vi "Gui.vi"() -> ()   [LabVIEW 2013]
uses:
  GlobalStop.vi
  GlobalWrite.vi
  GlobalMFC.vi
  GlobalGraph.vi
  GlobalMFCread.vi
panel:
  in  "TIME_INTERVAL (SECONDS)":dbl=1.0
  out "MFC_OUTPUT":dbl[](array[numeric])
  in  "MFC_INPUT":dbl[](array[numeric])
  out "URAS_OUTPUT_GRAPH":dynamicdata(graph)
  out "EUROTHERM_OUTPUT_GRAPH":dynamicdata(graph)
  in  "?":bool
  in  "EUROTHERM_INPUT":dbl[](array[numeric])
  out "EUROTHERM_OUTPUT":dbl[](array[numeric])
  # "O2"
  # "O2"
  # "CO"
  # "CO"
  # "HE"
  # "HE"
  # "N2"
  # "N2"
  # "CO2"
  # "CO2"
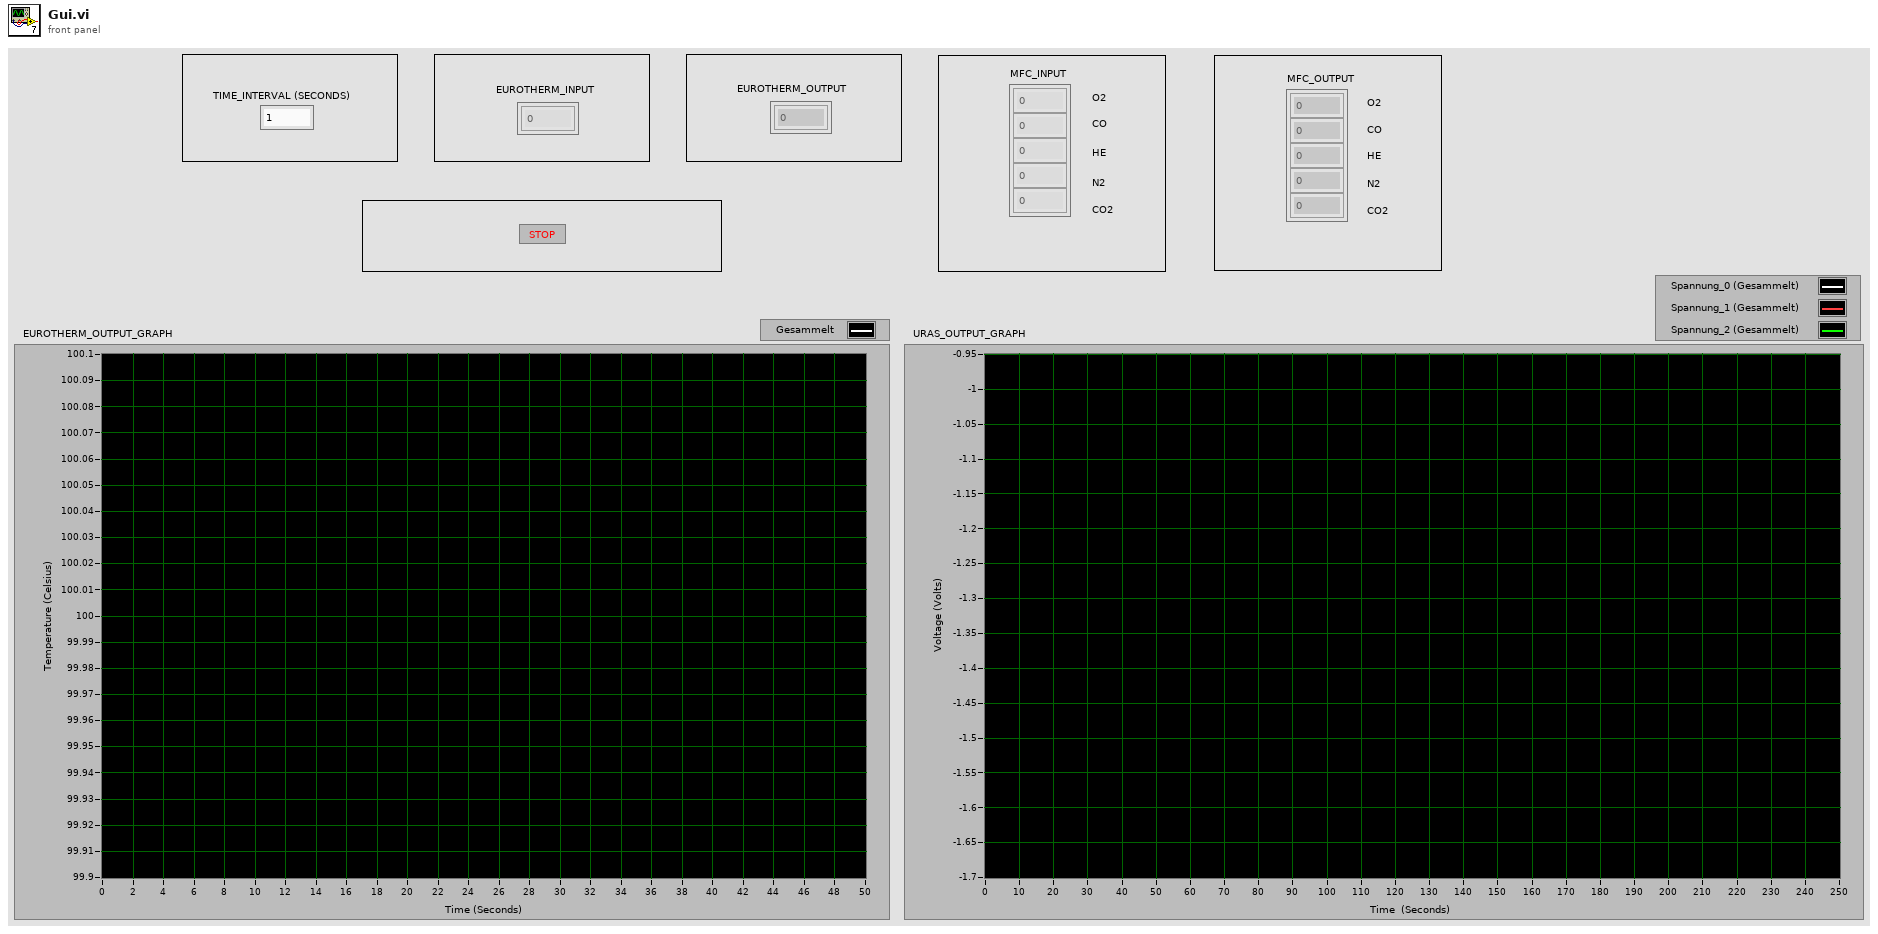
[diagram p1: front panel]
types:
  T1 = enum32{"Invalid", "Standard", "Closed", "Hidden", "Minimized", "Maximized"}
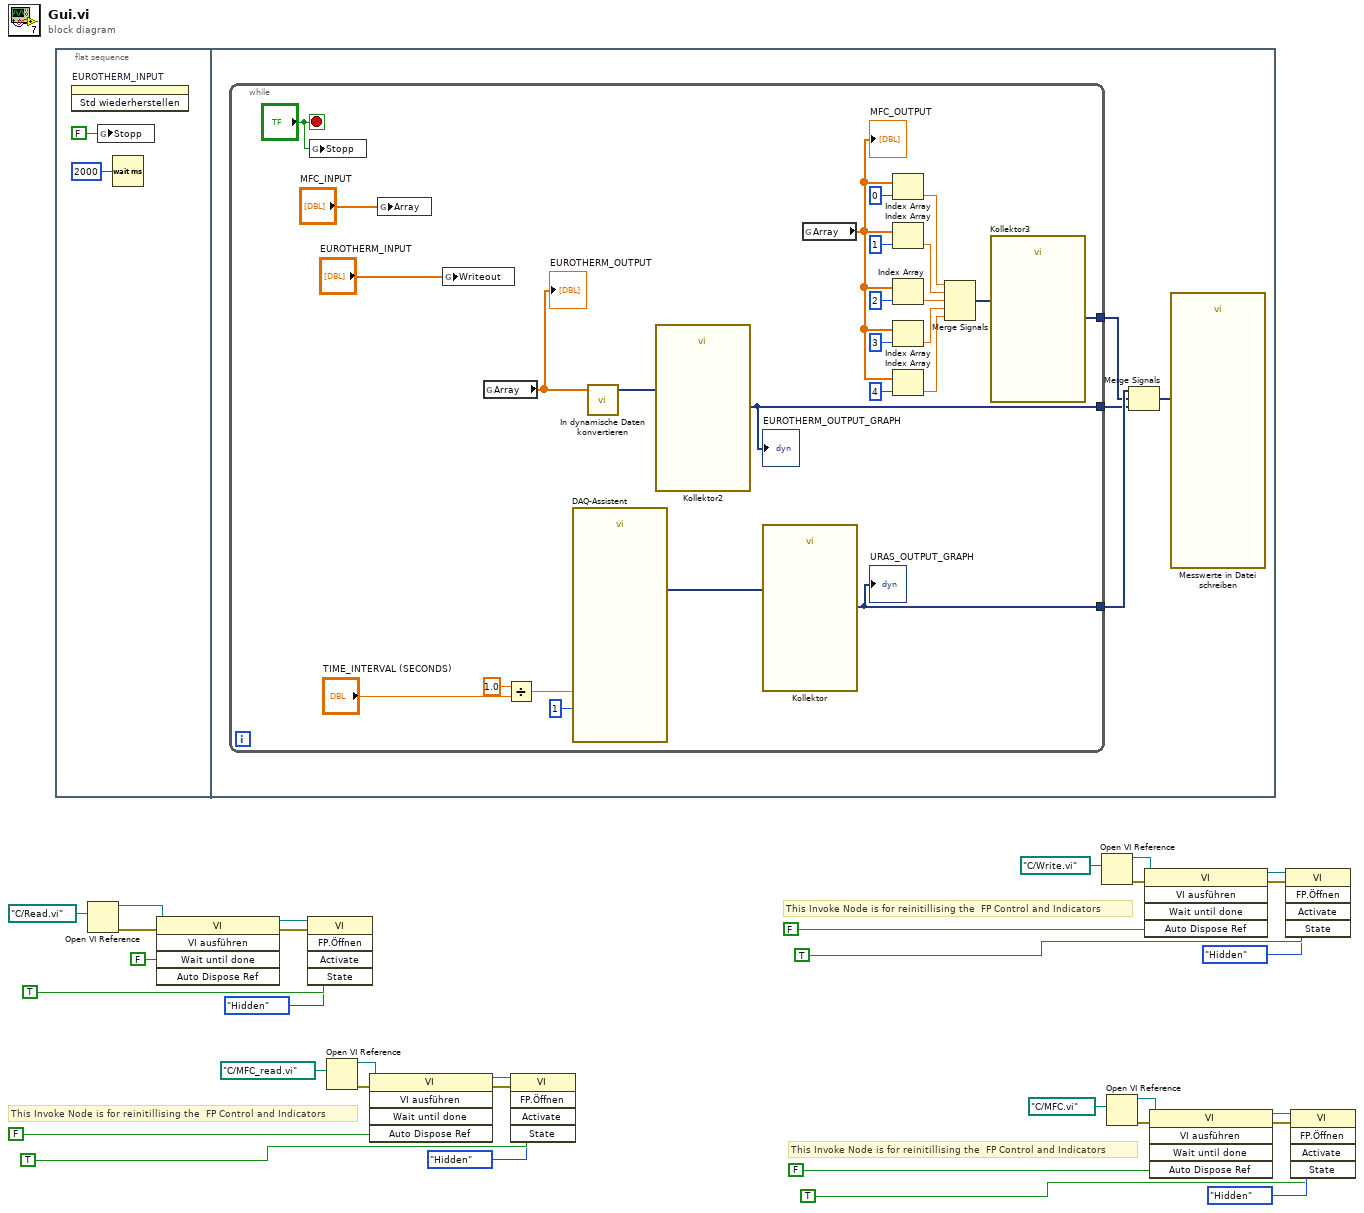
[diagram p0: block diagram]
diagram:
  # "This Invoke Node is for reinitillising the  FP Control and Indicators"
  # "This Invoke Node is for reinitillising the  FP Control and Indicators"
  # "This Invoke Node is for reinitillising the  FP Control and Indicators"
  n1 = flat-sequence {
    frame #0 {
      n2 = invoke on="EUROTHERM_INPUT" class="Arr (strikt)" method="Std wiederherstellen"() -> ()  [unwired: 3 in, 3 out]
      n3 = global write "GlobalStop.vi" "Stopp"(FALSE) -> ()
      n4 = Wait (ms)(milliseconds to wait=u32 2000 ("Zu wartende ms")) -> ()  [unwired: 1 out]
    }
    frame #1 {
      n5 = while {
        tunnel: [w60] -> w37
        tunnel: [w56] -> w35
        tunnel: [w51] -> w36
        stop <- "?" stop-if-true
        n6 = global write "GlobalStop.vi" "Stopp"("?") -> ()
        n7 = global write "GlobalMFC.vi" "Array"("MFC_INPUT") -> ()
        n8 = global write "GlobalWrite.vi" "Writeout"("EUROTHERM_INPUT") -> ()
        n9 = global read "GlobalGraph.vi" "Array"() -> (w50:dbl[])
        "EUROTHERM_OUTPUT" <- w50
        n10 = Divide(x=1.0, y="TIME_INTERVAL (SECONDS)") -> (x/y=w54:dbl)
        n11 = call "DAQ-Assistent"("Rate"=w54, "Sample-Anzahl"=1) -> ("data"=w61:dynamicdata)  [unwired: 14 in, 3 out]
        n12 = call "In dynamische Daten konvertieren"("Array"=w50) -> ("Dynamic Data Type"=w49:dynamicdata)  [unwired: 3 in]
        n13 = call "Kollektor2"("Signals"=w49) -> ("Collected Signals"=w51:dynamicdata)  [unwired: 9 in, 1 out]
        "EUROTHERM_OUTPUT_GRAPH" <- w51
        n14 = call "Kollektor"("Signals"=w61) -> ("Collected Signals"=w60:dynamicdata)  [unwired: 9 in, 1 out]
        "URAS_OUTPUT_GRAPH" <- w60
        n15 = global read "GlobalMFCread.vi" "Array"() -> (w48:dbl[])
        "MFC_OUTPUT" <- w48
        n16 = Index Array(array=w48, index=0 ("Index")) -> (element=w57:dbl)
        n17 = Index Array(array=w48, index=1 ("Index")) -> (element=w42:dbl)
        n18 = Index Array(array=w48, index=2 ("Index")) -> (element=w41:dbl)
        n19 = Index Array(array=w48, index=3 ("Index")) -> (element=w40:dbl)
        n20 = Index Array(array=w48, index=4 ("Index")) -> (element=w39:dbl)
        n21 = Merge Signals(w57, w42, w41, w40, w39) -> (w43:dynamicdata)
        n22 = call "Kollektor3"("Signals"=w43) -> ("Collected Signals"=w56:dynamicdata)  [unwired: 9 in, 1 out]
      }
      n23 = Merge Signals(w37, w35, w36) -> (w38:dynamicdata)
      n24 = call "Messwerte in Datei schreiben"("Signals"=w38) -> ()  [unwired: 16 in, 3 out]
    }
  }
  n25 = Open VI Reference(vi path=path "C:/Read.vi" ("VI-Pfad")) -> (vi reference=w29:refnum<vi>, error out=w28:errorcluster)  [unwired: 5 in]
  n26 = invoke class="VI" method="VI ausführen"(reference=w29, error in=w28, "Wait until done"=FALSE) -> (reference out=w24:refnum<vi>, error out=w23:errorcluster)  [unwired: 2 in, 3 out]
  n27 = invoke class="VI" method="FP.Öffnen"(reference=w24, error in=w23, "Activate"=TRUE ("Aktivieren?"), "State"=T1."Hidden" ("Zustand")) -> ()  [unwired: 1 in, 5 out]
  n28 = Open VI Reference(vi path=path "C:/MFC_read.vi" ("VI-Pfad")) -> (vi reference=w8:refnum<vi>, error out=w7:errorcluster)  [unwired: 5 in]
  n29 = invoke class="VI" method="VI ausführen"(reference=w8, error in=w7, "Wait until done"=FALSE) -> (reference out=w5:refnum<vi>, error out=w4:errorcluster)  [unwired: 2 in, 3 out]
  n30 = invoke class="VI" method="FP.Öffnen"(reference=w5, error in=w4, "Activate"=TRUE ("Aktivieren?"), "State"=T1."Hidden" ("Zustand")) -> ()  [unwired: 1 in, 5 out]
  n31 = Open VI Reference(vi path=path "C:/Write.vi" ("VI-Pfad")) -> (vi reference=w32:refnum<vi>, error out=w31:errorcluster)  [unwired: 5 in]
  n32 = Open VI Reference(vi path=path "C:/MFC.vi" ("VI-Pfad")) -> (vi reference=w10:refnum<vi>, error out=w11:errorcluster)  [unwired: 5 in]
  n33 = invoke class="VI" method="VI ausführen"(reference=w32, error in=w31, "Wait until done"=FALSE) -> (reference out=w20:refnum<vi>, error out=w19:errorcluster)  [unwired: 2 in, 3 out]
  n34 = invoke class="VI" method="VI ausführen"(reference=w10, error in=w11, "Wait until done"=FALSE) -> (reference out=w13:refnum<vi>, error out=w14:errorcluster)  [unwired: 2 in, 3 out]
  n35 = invoke class="VI" method="FP.Öffnen"(reference=w20, error in=w19, "Activate"=TRUE ("Aktivieren?"), "State"=T1."Hidden" ("Zustand")) -> ()  [unwired: 1 in, 5 out]
  n36 = invoke class="VI" method="FP.Öffnen"(reference=w13, error in=w14, "Activate"=TRUE ("Aktivieren?"), "State"=T1."Hidden" ("Zustand")) -> ()  [unwired: 1 in, 5 out]
